vi "Configure Alarm Hysteresis Math.vi"(0 "VISA resource name":refnum<visa-resource-name>, 5 "Math Channel (001)":string="001", 7 "Alarm No. (1)":i32=1 min=1 max=4, 9 "Measurement Channel Hysteresis (0)":i32 min=0 max=100000 step=1, 11 "error in (no error)":errorcluster) -> (4 "VISA resource name out":refnum<visa-resource-name>, 6 "Math Channel":string, 8 "Alarm No.":i32, 15 "error out":errorcluster)   [LabVIEW 2020, in "Yokogawa GX Series.lvlib"]
doc: "Sets the alarm hysteresis of a math channel.\n\nCommand: SAlmHysMath"
uses:
  <instrlib>/Yokogawa GX Series/Yokogawa GX Series.lvlib
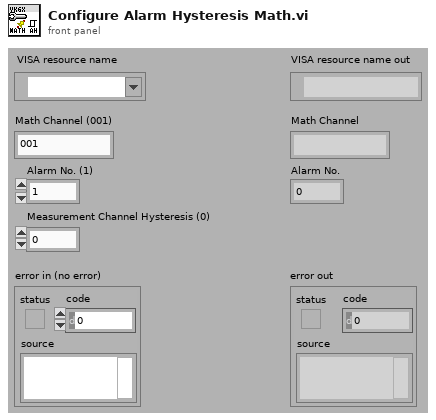
[diagram p1: front panel]
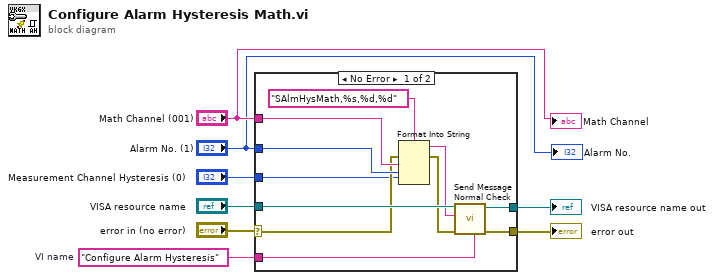
[diagram p0: block diagram]
diagram:
  w7 = "Configure Alarm Hysteresis"  # VI name
  n1 = case shown="No Error" "error in (no error)" {
    selector: "error in (no error)" -> [w10 w20]
    tunnel: "VISA resource name" -> [w18 w21]
    tunnel: w7 -> [w15 _]
    tunnel: "Math Channel (001)" -> [w14 _]
    tunnel: "Alarm No. (1)" -> [w13 _]
    tunnel: "Measurement Channel Hysteresis (0)" -> [w9 _]
    tunnel: [w12 w21] -> w5
    tunnel: [w11 w20] -> w4
    frame No Error {
      n2 = Format Into String(format string="SAlmHysMath,%s,%d,%d", error in=w10, w14, w13, w9) -> (resulting string=w16:string, error out=w17:errorcluster)  [unwired: 1 in]
      n3 = call <instrlib>:"Send Message Normal Check.vi"("Source (\"\")"=w15, "error in (no error)"=w17, "Send Message (\"\")"=w16, "VISA resource name"=w18) -> ("error out"=w11:errorcluster, "VISA resource name out"=w12:refnum<visa-resource-name>)  [unwired: 2 in, 4 out]
    }
    frame Error {
    }
  }
  "error out" <- w4
  "VISA resource name out" <- w5
  "Math Channel" <- "Math Channel (001)"
  "Alarm No." <- "Alarm No. (1)"
